vi "FG COP Map.vi"(1 "FG Action (Read)":T1, 2 "Map in":cluster{"Y":dbl[], "X":dbl[]}) -> (0 "Map out":cluster{"Y":dbl[], "X":dbl[]})   [LabVIEW 2011]
uses:
  cRIO/Functional Global Variables/Actions for FG's.ctl
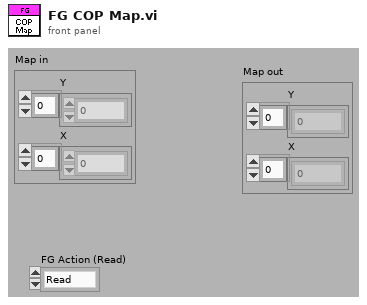
[diagram p1: front panel]
types:
  T1 = typedef "Actions for FG's.ctl" = enum16{"Read", "Write"}
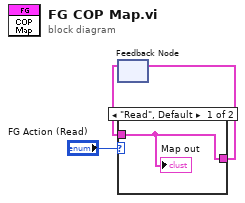
[diagram p0: block diagram]
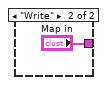
[diagram p2: hidden frame]
diagram:
  n1 = feedback #1() -> (w1:cluster{"Y":dbl[], "X":dbl[]})  [unwired: 1 in]
  n2 = case shown="\"Read\", Default" "FG Action (Read)" {
    tunnel: [w4 "Map in"] -> w2
    tunnel: w1 -> [w4 _]
    frame "Read", Default {
      "Map out" <- w4
    }
    frame "Write" {
    }
  }
  n3 = feedback-in #1(w2) -> ()
